vi "MatrixDUTSwitch.vi"(8 "error in (no error)":errorcluster, 10 "DUT #":i32, 11 "Switching in":refnum<class "Switching.lvclass">) -> (0 "error out":errorcluster, 3 "Switching out":refnum<class "Switching.lvclass">)   [LabVIEW 2013, in "Switching.lvclass"]
uses:
  Switching.lvclass
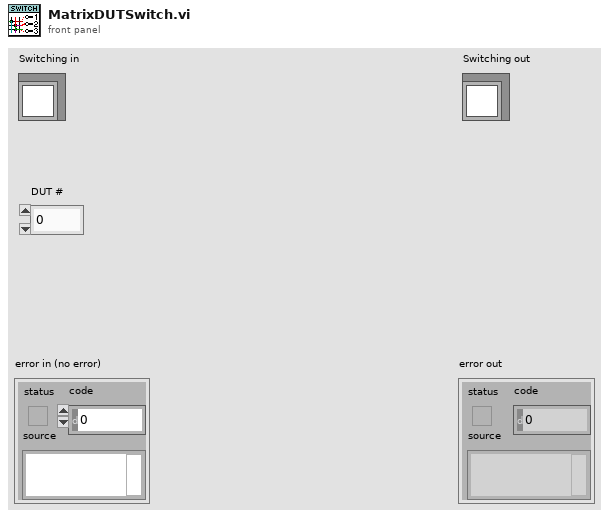
[diagram p1: front panel]
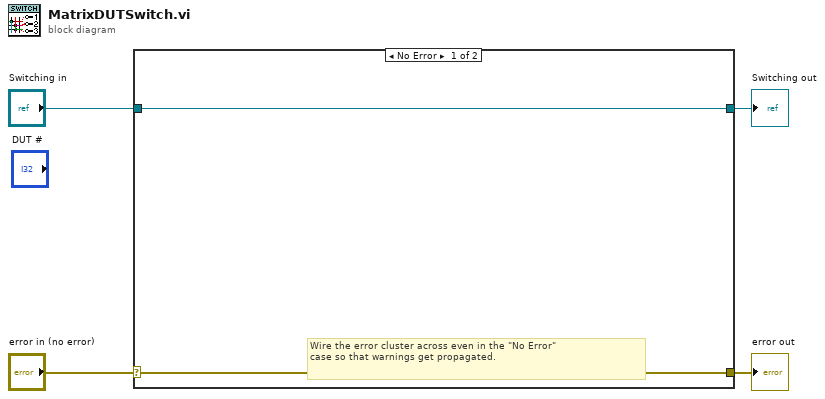
[diagram p0: block diagram]
diagram:
  n1 = case shown="No Error" "error in (no error)" {
    selector: "error in (no error)" -> [w5 w8]
    tunnel: [w5 w8] -> w3
    tunnel: [w6 w7] -> w1
    tunnel: "Switching in" -> [w6 w7]
    frame No Error {
      # "Wire the error cluster across even in the \"No Error\"\ncase so that warnings get propagated."
    }
    frame Error {
    }
  }
  "error out" <- w3
  "Switching out" <- w1
